vi "reset_command_queue.vi"(8 "error in (no error)":errorcluster, 11 "GenericToplevelComponent in":refnum<class "GenericToplevelComponent.lvclass">) -> (0 "error out":errorcluster, 2 "remaining commands":refnum<class "GenericCommand.lvclass">[](array[class]), 3 "GenericToplevelComponent out":refnum<class "GenericToplevelComponent.lvclass">)   [LabVIEW 2010, in "GenericToplevelComponent.lvclass"]
uses:
  GenericToplevelComponent.lvclass
  components/Command/GenericCommand/GenericCommand/GenericCommand.lvclass
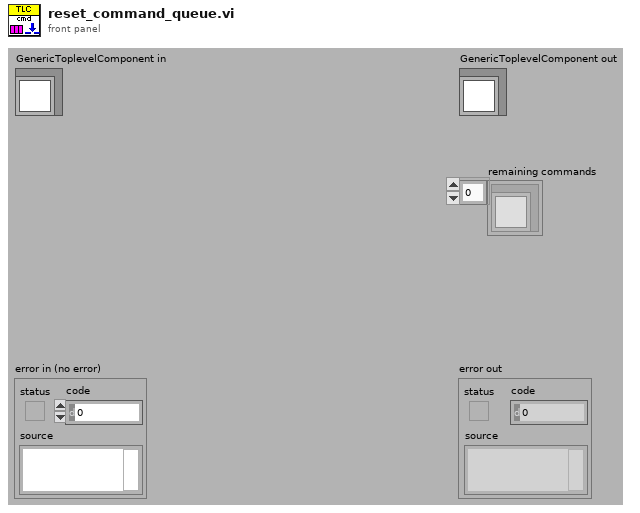
[diagram p1: front panel]
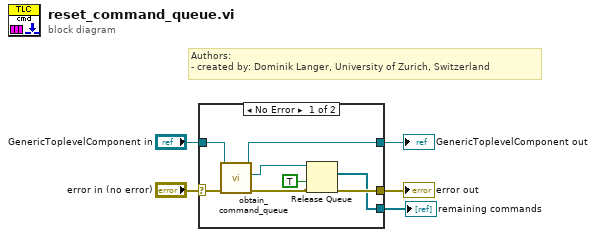
[diagram p0: block diagram]
diagram:
  # "Authors: \n- created by: Dominik Langer, University of Zurich, Switzerland"
  n1 = case shown="No Error" "error in (no error)" {
    selector: "error in (no error)" -> [w11 w15]
    tunnel: [w10 w15] -> w4
    tunnel: [w12 w14] -> w2
    tunnel: "GenericToplevelComponent in" -> [w13 w14]
    tunnel: [w9 _] -> w1
    frame No Error {
      n2 = call-dynamic "obtain_command_queue.vi"("error in (no error)"=w11, "GenericToplevelComponent in"=w13) -> ("error out"=w8:errorcluster, "command queue"=w7:refnum<queue>, "GenericToplevelComponent out"=w12:refnum<class "GenericToplevelComponent.lvclass">)  [unwired: 7 in]
      n3 = Release Queue(queue=w7, force destroy? (F)=TRUE, error in (no error)=w8) -> (remaining elements=w9:refnum<class "GenericCommand.lvclass">[], error out=w10:errorcluster)  [unwired: 1 out]
    }
    frame Error {
    }
  }
  "error out" <- w4
  "GenericToplevelComponent out" <- w2
  "remaining commands" <- w1
